vi "PCO_GetTemperature.vi"(0 "ph":u64, 11 "error in (no error)":errorcluster {"code" format="%x"}) -> (3 "sCamTemp":i16, 4 "ph out":u64, 6 "ErrorMessage":i32 format="%x", 8 "sCCDTemp":dbl, 14 "sPowTemp":i16, 15 "error out":errorcluster {"code" format="%x"})   [LabVIEW 2020, in "SDK.lvlib" / "GeneralCameraStatus.lvlib"]
doc: "<b>Description:</b>\nThis function retrieves the current temperatures in °C of the imaging sensor, camera and additional devices e.g. power supply. The image sensor and the additional device temperature are not available for all cameras. In this case the following values will be returned:\nImage sensor temperature missing: sCCDTemp = 0x8000\nAdditional device temperature missing: sPowTemp = 0x0000\n\n<b>Supported camera type:</b>\nAll cameras\n\n<b>Descriptor dependency:</b>\nNone"
uses:
  GeneralCameraStatus.lvlib
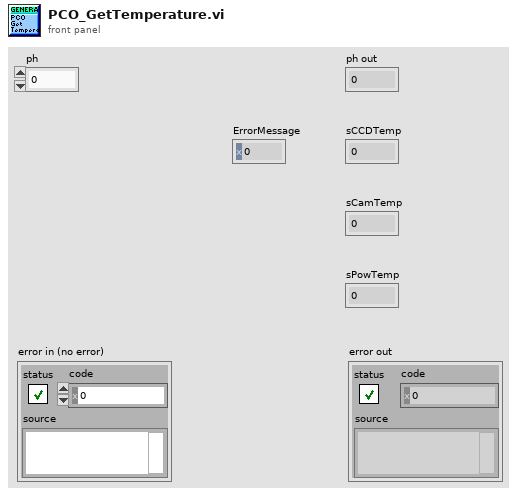
[diagram p1: front panel]
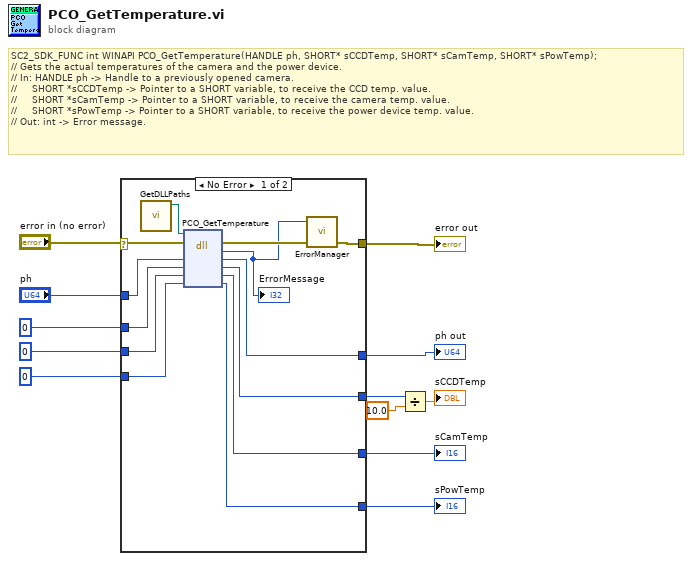
[diagram p0: block diagram]
diagram:
  # "SC2_SDK_FUNC int WINAPI PCO_GetTemperature(HANDLE ph, SHORT* sCCDTemp, SHORT* sCamTemp, SHORT* sPowTemp);\n// Gets the actual temperatures of the camera and the power device.\n// In: HANDLE ph -> Handle to a previously opened camera.\n//     SHORT *sCCDTemp -> Pointer to a SHORT variable, to receive the CCD temp. value.\n//     SHORT *sCamTemp -> Pointer to a SHORT variable, to receive the camera temp. value.\n//     SHORT *sPowTemp -> Pointer to a SHORT variable, to receive the power device temp. value.\n// Out: int -> Error message."
  n1 = case shown="No Error" "error in (no error)" {
    selector: "error in (no error)" -> [w21 w30]
    tunnel: "ph" -> [w25 w29]
    tunnel: [w23 w30] -> w11
    tunnel: [w20 w29] -> w9
    tunnel: i16 0 ("sCCDTemp") -> [w19 w28]
    tunnel: i16 0 ("sCCDTemp") -> [w18 w27]
    tunnel: i16 0 ("sCCDTemp") -> [w17 w26]
    tunnel: [w16 w28] -> w3
    tunnel: [w15 w26] -> w2
    tunnel: [w14 w27] -> w1
    frame No Error {
      n2 = call "GetDLLPaths.vi"() -> ("SC2_Cam_Path"=w13:path)  [unwired: 9 in, 2 out]
      n3 = dll-call lib="?" fn="PCO_GetTemperature"(path in=w13, error in=w21, "ph"=w25, "sCCDTemp"=w19, "sCamTemp"=w18, "sPowTemp"=w17) -> (error out=w24:errorcluster, "return type"=w22:i32, "ph"=w20:u64, "sCCDTemp"=w16:i16, "sCamTemp"=w14:i16, "sPowTemp"=w15:i16)  [unwired: 1 in, 1 out]
      "ErrorMessage" <- w22
      n4 = call "ErrorManager.vi"("error in (no error)"=w24, "error code"=w22) -> ("error out"=w23:errorcluster)  [unwired: 3 in]
    }
    frame Error {
    }
  }
  "error out" <- w11
  "ph out" <- w9
  "sCamTemp" <- w1
  "sPowTemp" <- w2
  n5 = Divide(x=w3, y=sgl 10.0) -> (x/y=→"sCCDTemp":sgl)
